vi "AgNA_Get Trace.vi"(0 "Network Analyzer":refnum<k15>, 1 "Apply Calibration":bool, 2 "S21(True)_S12(False)":bool, 3 "Val":dbl=-20.0 format="%#_13g", 5 "Calset Name (\"D:\\user\\data\")":string="D:\\user\\data" caption="File Name (\"D:\\user\\data\")", 7 "Stop":dbl, 9 "Start":dbl, 11 "error in":errorcluster, 12 "Number of Points":i32=2401) -> (4 "Magnitude Trace":dbl[](array[numeric]), 6 "Frequency Trace":dbl[](array[numeric]) caption="Trace Data" format="%^.3e", 15 "error out":errorcluster {"code" format="%.0x"})   [LabVIEW 2015]
uses:
  <instrlib>/Agilent NA/Agilent NA.lvlib
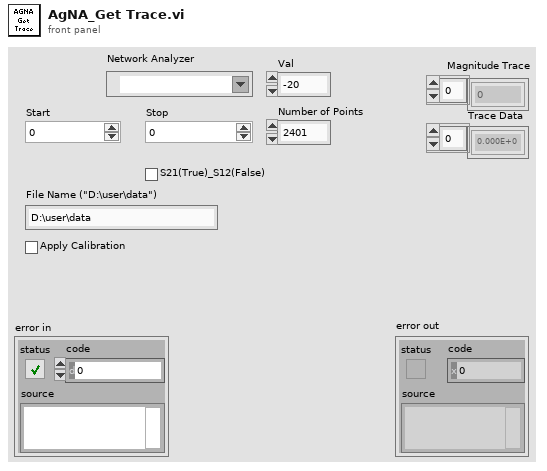
[diagram p1: front panel]
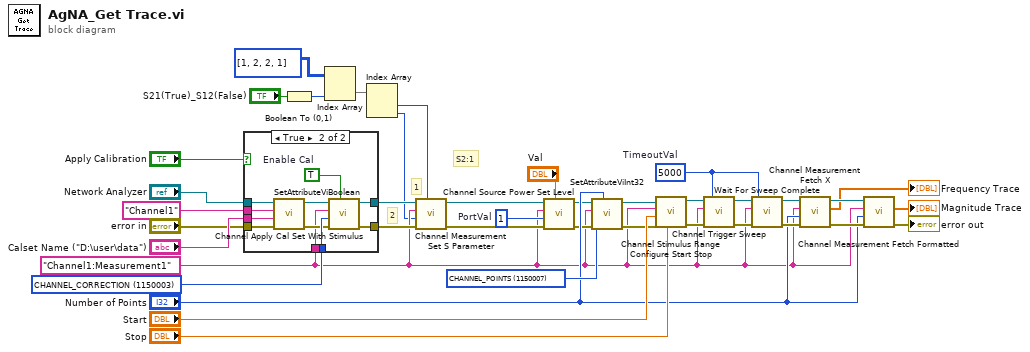
[diagram p0: block diagram]
diagram:
  w14 = 1  # PortVal
  w21 = u32 1150007 items=["CHANNEL_AVERAGING_FACTOR"=1150002, "CHANNEL_MEASUREMENT_ELECTRICAL_DELAY_MEDIUM"=1150178, "CHANNEL_MEASUREMENT_ELECTRICAL_DELAY_UNITS"=1150175, "CHANNEL_MEASUREMENT_FORMAT"=1150014, "CHANNEL_MEASUREMENT_LIMIT_NUMBER"=1150020, "CHANNEL_MEASUREMENT_TIME_DOMAIN_GATING_SHAPE"=1150140, "CHANNEL_MEASUREMENT_TIME_DOMAIN_GATING_TYPE"=1150144, "CHANNEL_MEASUREMENT_TIME_DOMAIN_PARAMETERS"=1150137, "CHANNEL_MEASUREMENT_TIME_DOMAIN_TRANSFORM_MODE"=1150147, "CHANNEL_MEASUREMENT_TRACE_MATH"=1150017, "CHANNEL_POINTS"=1150007, "CHANNEL_SWEEP_MODE"=1150009, "CHANNEL_SWEEP_TYPE"=1150012, "CHANNEL_TRIGGER_MODE"=1150013, "DISPLAY_ARRANGE_WINDOWS"=1150181, "SYSTEM_TIME_OUT_MILLISECONDS"=1150040, "TRIGGER_SOURCE"=1150042, "WINDOW_SIZE"=1150133, "WINDOW_TABLE"=1150134] ("AttributeID")
  w23 = 5000  # TimeoutVal
  w7 = "Channel1:Measurement1" ("RepCapIdentifier")
  w38 = u32 1150003 items=["CHANNEL_AVERAGING"=1150001, "CHANNEL_CORRECTION"=1150003, "CHANNEL_MEASUREMENT_LIMIT_ENABLE"=1150018, "CHANNEL_MEASUREMENT_MARKER_ENABLED"=1150022, "CHANNEL_MEASUREMENT_MARKER_MARKER_TRACK_ENABLED"=1150023, "CHANNEL_MEASUREMENT_SMOOTHING"=1150015, "CHANNEL_MEASUREMENT_TIME_DOMAIN_COUPLING_STATE"=1150136, "CHANNEL_MEASUREMENT_TIME_DOMAIN_GATING_ENABLE"=1150139, "CHANNEL_MEASUREMENT_TIME_DOMAIN_TRANSFORM_ENABLE"=1150146, "CHANNEL_MEASUREMENT_TRACE_ENABLE_TRACE_MAX"=1150182, "CHANNEL_PORT_EXTENSION_STATUS"=1150008, "CHANNEL_SOURCEPOWER_COUPLING"=1150031, "CHANNEL_SWEEP_TIME_AUTO"=1150011, "DISPLAY_ENABLED"=1150036, "GUIDED_CALIBRATION_ADVANCED_E_CAL_AUTO_ORIENTATION"=1150116, "SIMULATE"=1050005, "SYSTEM_POWER_ENABLED"=1150184, "SYSTEM_TRACE_ENABLED"=1150041, "WINDOW_STATE"=1150183, "WINDOW_TITLE_STATE"=1150132] ("AttributeID")
  # "2"
  # "1"
  # "S2:1"
  n1 = case shown="True" "Apply Calibration" {
    tunnel: "Channel1" ("Channel") -> [_ w52]
    tunnel: w38 -> [_ w51]
    tunnel: "Calset Name (\"D:\\user\\data\")" -> [_ w47]
    tunnel: [w40 w46] -> w11
    tunnel: [w41 w45] -> w10
    tunnel: "error in" -> [w41 w44]
    tunnel: "Network Analyzer" -> [w40 w43]
    tunnel: w7 -> [_ w42]
    frame False {
    }
    frame True {
      w49 = TRUE  # Enable Cal
      n2 = call <instrlib>:"Channel Apply Cal Set With Stimulus.vi"("error in (no error)"=w44, "CalSetName"=w47, "Channel"=w52, "instrument handle"=w43) -> ("error out"=w48:errorcluster, "instrument handle out"=w50:refnum<k15>)  [unwired: 6 in]
      n3 = call <instrlib>:"SetAttributeViBoolean.vi"("AttributeValue (Off)"=w49, "error in (no error)"=w48, "AttributeID"=w51, "RepCapIdentifier"=w42, "instrument handle"=w50) -> ("error out"=w45:errorcluster, "instrument handle out"=w46:refnum<k15>)  [unwired: 5 in]
    }
  }
  n4 = Boolean To (0,1)(Boolean="S21(True)_S12(False)") -> (0, 1=w4:i16)
  n5 = Index Array(array=i32[][] [[1, 2], [2, 1]], index (col)=w4) -> (element=w3:i32[])  [unwired: 1 in]
  n6 = Index Array(array=w3) -> (element #1=w2:i32, element #2=w1:i32)  [unwired: 2 in]
  n7 = call <instrlib>:"Channel Measurement Set S Parameter.vi"("NewSourcePortVal"=w2, "error in (no error)"=w10, "NewReceiverPortVal"=w1, "RepCapIdentifier"=w7, "instrument handle"=w11) -> ("error out"=w9:errorcluster, "instrument handle out"=w8:refnum<k15>)  [unwired: 5 in]
  n8 = call <instrlib>:"Channel Source Power Set Level.vi"("Val"="Val", "error in (no error)"=w9, "PortVal"=w14, "RepCapIdentifier"=w7, "instrument handle"=w8) -> ("error out"=w17:errorcluster, "instrument handle out"=w16:refnum<k15>)  [unwired: 5 in]
  n9 = call <instrlib>:"SetAttributeViInt32.vi"("AttributeValue"="Number of Points", "error in (no error)"=w17, "AttributeID"=w21, "RepCapIdentifier"=w7, "instrument handle"=w16) -> ("error out"=w19:errorcluster, "instrument handle out"=w20:refnum<k15>)  [unwired: 5 in]
  n10 = call <instrlib>:"Channel Stimulus Range Configure Start Stop.vi"("StopVal"="Stop", "error in (no error)"=w19, "StartVal"="Start", "RepCapIdentifier"=w7, "instrument handle"=w20) -> ("error out"=w25:errorcluster, "instrument handle out"=w24:refnum<k15>)  [unwired: 5 in]
  n11 = call <instrlib>:"Channel Trigger Sweep.vi"("error in (no error)"=w25, "TimeoutVal"=w23, "RepCapIdentifier"=w7, "instrument handle"=w24) -> ("error out"=w26:errorcluster, "instrument handle out"=w29:refnum<k15>)  [unwired: 6 in]
  n12 = call <instrlib>:"Wait For Sweep Complete.vi"("error in (no error)"=w26, "MaxTimeMilliseconds"=w23, "Channel"=w7, "instrument handle"=w29) -> ("error out"=w28:errorcluster, "instrument handle out"=w27:refnum<k15>)  [unwired: 6 in]
  n13 = call <instrlib>:"Channel Measurement Fetch X.vi"("error in (no error)"=w28, "RetValBufferSize"="Number of Points", "RepCapIdentifier"=w7, "instrument handle"=w27) -> ("error out"=w35:errorcluster, "RetVal"=→"Frequency Trace":dbl[], "instrument handle out"=w36:refnum<k15>)  [unwired: 4 in, 1 out]
  n14 = call <instrlib>:"Channel Measurement Fetch Formatted.vi"("error in (no error)"=w35, "RetValBufferSize"="Number of Points", "RepCapIdentifier"=w7, "instrument handle"=w36) -> ("error out"=→"error out":errorcluster, "RetVal"=→"Magnitude Trace":dbl[])  [unwired: 4 in, 2 out]
